vi "GetSystemTime.vi"(0 "As UTC?":bool=TRUE caption="As UTC? (T)", 11 "Error in":errorcluster caption="Error in (no error)") -> (4 "Time and Date":T1, 15 "Error out":errorcluster)   [LabVIEW 2017, in "GPTiming.lvlib"]
doc: "Gets the current system <B>Time and Date</B>.\n\nThis VI queries Windows for the time and date (<B>thus this VI is Windows only</B>). Since LabVIEW does not register if the time zone has changed at runtime, this VI can be necessary in applications where the time, date and/or timezone is changed manually or programmatically at runtime.\n\nIf <B>As UTC?</B> is True (default) the time is returned in UTC time. If <B>As UTC?</B> is False the time is returned in the local system time zone and DST observation.\n\nThis VI runs only if there is no error on <B>Error in</B>.\n\nSteen Schmidt\nGPower\n4/2 2017"
uses:
  GPTiming.lvlib
  kernel32.dll
  Date.ctl
  Time.ctl
  TimeAndDate.ctl
  Error/GPError.lvlib
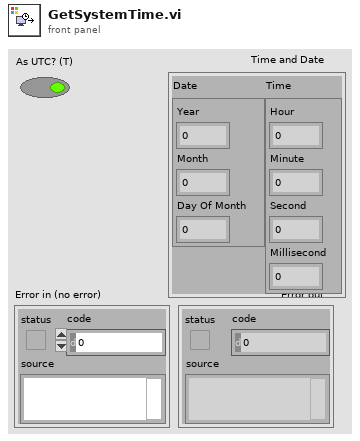
[diagram p1: front panel]
types:
  T1 = typedef "GPTiming.lvlib/TimeAndDate.ctl" = cluster{"Date":T2, "Time":T3}
  T2 = typedef "GPTiming.lvlib/Date.ctl" = cluster{"Year":u16, "Month":u16, "Day Of Month":u16}
  T3 = typedef "GPTiming.lvlib/Time.ctl" = cluster{"Hour":u16, "Minute":u16, "Second":u16, "Millisecond":u16}
  T4 = cluster{"Year":u16, "Month":u16, "Day of Week":u16, "Day of Month":u16, "Hour":u16, "Minute":u16, "Second":u16, "Millisecond":u16}
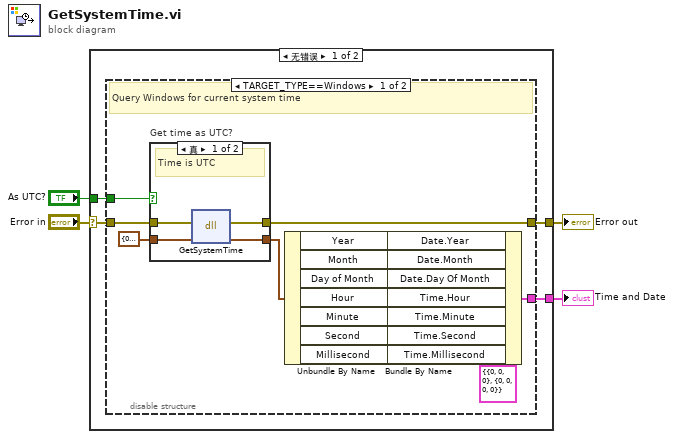
[diagram p0: block diagram]
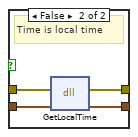
[diagram p2: hidden frame]
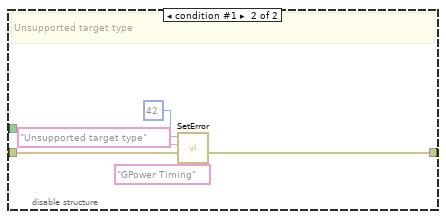
[diagram p3: hidden frame]
diagram:
  n1 = case shown="无错误" "Error in" {
    selector: "Error in" -> [w8 w36]
    tunnel: [w7 w36] -> w3
    tunnel: [w6 _] -> w4
    tunnel: "As UTC?" -> [w5 _]
    frame No Error {
      n2 = disable-structure shown="TARGET_TYPE==Windows" {
        disable-tunnel: w8 -> [w12 w33]
        disable-tunnel: [w11 w31] -> w7
        disable-tunnel: [w10 _] -> w6
        disable-tunnel: w5 -> [w9 _]
        frame condition #0 (active) {
          # "Query Windows for current system time"
          n3 = case "Get time as UTC?" shown="真" w9 {
            tunnel: T4 {"Year"=0, "Month"=0, "Day of Week"=0, "Day of Month"=0, "Hour"=0, "Minute"=0, "Second"=0, "Millisecond"=0} ("System Time") -> [w26 w30]
            tunnel: w12 -> [w25 w29]
            tunnel: [w24 w28] -> w11
            tunnel: [w23 w27] -> w14
            frame True {
              # "Time is UTC"
              n4 = dll-call lib="kernel32.dll" fn="GetSystemTime"(error in=w25, "Time"=w26) -> (error out=w24:errorcluster, "Time"=w23:T4)  [unwired: 3 in, 1 out]
            }
            frame False {
              # "Time is local time"
              n5 = dll-call lib="kernel32.dll" fn="GetLocalTime"(error in=w29, "Time"=w30) -> (error out=w28:errorcluster, "Time"=w27:T4)  [unwired: 3 in, 1 out]
            }
          }
          n6 = Unbundle By Name(w14) -> ("Year"=w16:u16, "Month"=w17:u16, "Day of Month"=w18:u16, "Hour"=w19:u16, "Minute"=w20:u16, "Second"=w21:u16, "Millisecond"=w22:u16)
          n7 = Bundle By Name(cluster=T1 {"Date"={"Year"=0, "Month"=0, "Day Of Month"=0}, "Time"={"Hour"=0, "Minute"=0, "Second"=0, "Millisecond"=0}} ("Date & Time"), "Date.Year"=w16, "Date.Month"=w17, "Date.Day Of Month"=w18, "Time.Hour"=w19, "Time.Minute"=w20, "Time.Second"=w21, "Time.Millisecond"=w22) -> (w10:T1)
        }
        frame condition #1 {
          # "Unsupported target type"
          n8 = call "SetError.vi"("Error label"="GPower Timing", "Error in"=w33, "Error description"="Unsupported target type", "Error code"=42) -> ("Error out"=w31:errorcluster)  [unwired: 7 in]
        }
      }
    }
    frame Error {
    }
  }
  "Error out" <- w3
  "Time and Date" <- w4
